vi "NumIntegrate_Rkdp_impl.vi"(4 "MaxTruncError":dbl, 5 "Func_X_U_Extra":T1, 6 "dT_Remaining":dbl, 7 "PassedData":variant, 8 "InitialH":dbl, 10 "U":T2, 11 "X":T2) -> (0 "Error":bool, 1 "IterationCount":i32, 2 "H":dbl, 3 "NewX":T2)   [LabVIEW 2019, in "Trajectory_Library.lvlib"]
doc: "Implements one loop of RKDP. This takes an initial state, dt guess, and max truncation error, and returns a new x and the dt over which that x was updated. This should be called until there is no dt remaining.\n\nThis is an INTERNAL FUNCTION AND SHOULD NOT BE CALLED DIRECTLY.\n\n\n\nInputs:\n - Func_X_U_Extra -- A strictly typed LabVIEW reference to a function to integrate as a function of matrix X, U, and the extra passed data\n - PassedData -- This is a variant that can be used to pass additional data to the function if needed. The data must be packed into the variant in the specific way expected by the function.\n - X -- The initial value of x.\n - U -- The value u held constant over the integration period.\n - InitialH -- The initial dt guess. This is refined to clamp truncation error to the specified max.\n - dT_Remaining -- How much time is left to integrate over. Used to clamp h.\n - Max TruncError -- The max truncation error acceptable. Usually a small number like 1e-6.\n\nOutputs:\n - New X -- the integration of dx/dt = f(x, u) for dt\n - H -- \n - Iteration count -- How many times this routine looped to achieve the desired error tolerance\n - Error -- If TRUE, an error occured."
uses:
  Trajectory_Library.lvlib
  <vilib>/Analysis/Matrix/Datatypes/RealMatrix.ctl
  TypeDef/CALLBACK_FUNC_TYPE.ctl
  NumIntegrate_Rkdp_Func_B1.vi
  NumIntegrate_Rkdp_Func_B2.vi
  <vilib>/Analysis/_algsub.llb/Matrix Norm.vi
  <vilib>/Analysis/_algsub.llb/Real Matrix Norm.vi
  <vilib>/Analysis/Matrix/Numeric/Multiply/Multiply - RM,R.vi
  <vilib>/Analysis/Matrix/Numeric/Add/Add - RM,RM.vi
  <vilib>/Analysis/Matrix/NI_Matrix.lvlib
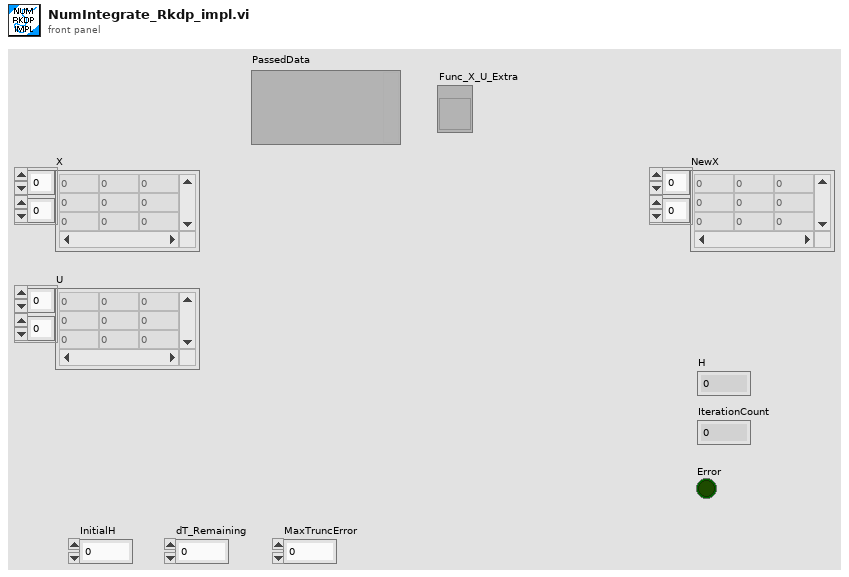
[diagram p1: front panel]
types:
  T1 = typedef "Trajectory_Library.lvlib/CALLBACK_FUNC_TYPE.ctl" = refnum<vi>
  T2 = typedef "NI_Matrix.lvlib/RealMatrix.ctl" = dbl[][]
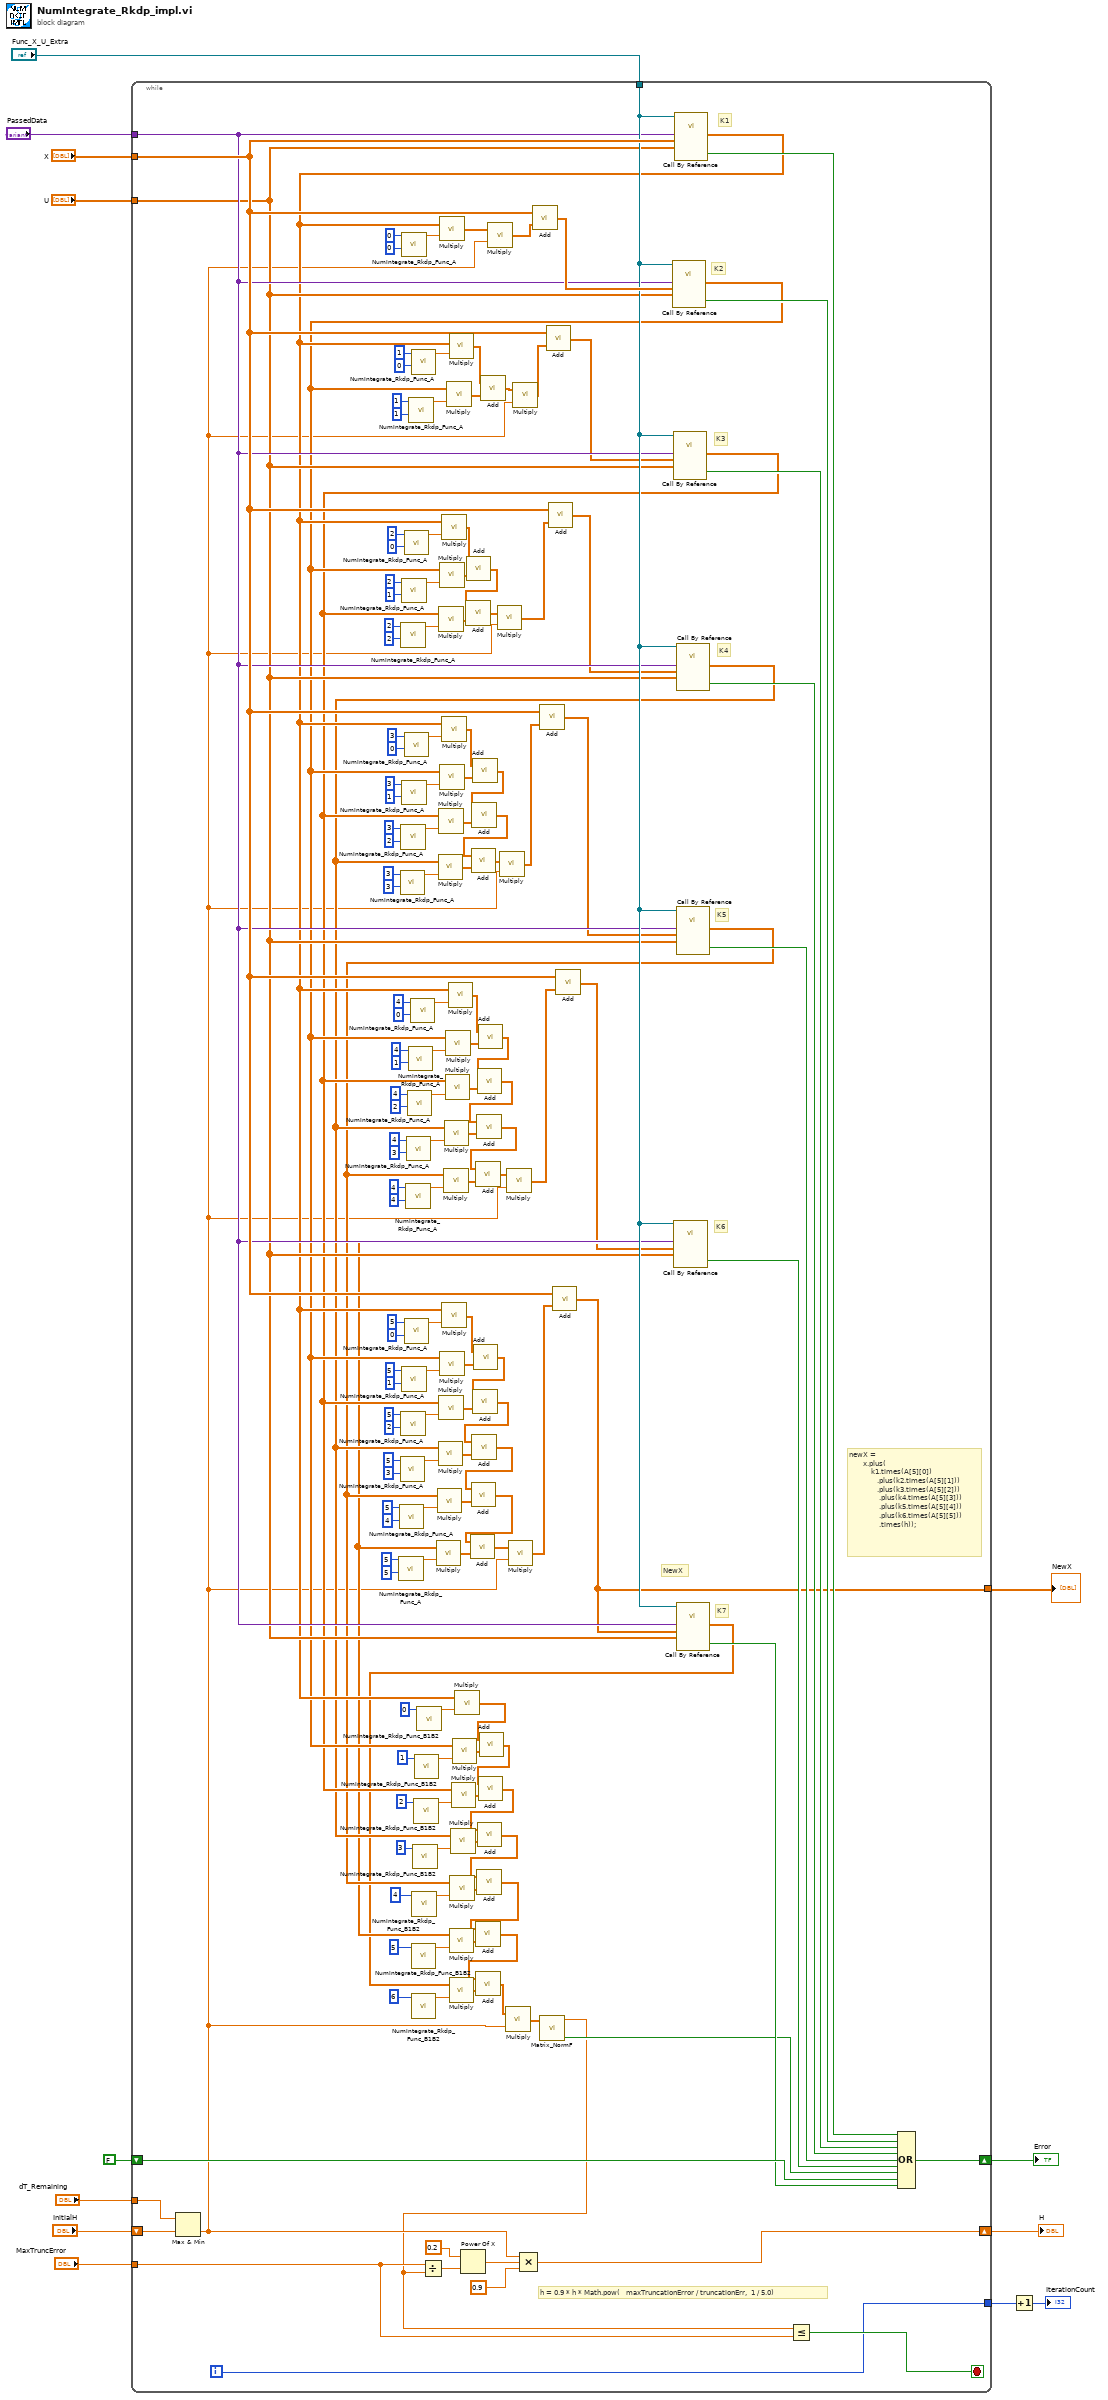
[diagram p0: block diagram]
diagram:
  n1 = while {
    tunnel: "PassedData" -> [w54]
    shift-right: [w76] -> w8
    shift-left: "InitialH" -> [w75]
    tunnel: "X" -> [w70]
    tunnel: "U" -> [w53]
    tunnel: "MaxTruncError" -> [w73]
    tunnel: "dT_Remaining" -> [w74]
    tunnel: [w24] -> w5
    tunnel: [w71] -> w7
    tunnel: "Func_X_U_Extra" -> [w55]
    shift-right: [w62] -> w1
    shift-left: FALSE -> [w69]
    i -> [w71]
    stop <- w72 stop-if-true
    # "K7"
    # "newX =\n       x.plus(\n           k1.times(A[5][0])\n              .plus(k2.times(A[5][1]))\n              .plus(k3.times(A[5][2]))\n               .plus(k4.times(A[5][3]))\n               .plus(k5.times(A[5][4]))\n               .plus(k6.times(A[5][5]))\n               .times(h));"
    # "K6"
    # "K5"
    # "K4"
    # "K3"
    # "K2"
    # "K1"
    # "h = 0.9 * h * Math.pow(   maxTruncationError / truncationErr,  1 / 5.0)"
    # "NewX"
    n2 = Max & Min(x=w74, y=w75) -> (min(x,y)=w17:dbl)  [unwired: 1 out]
    n3 = call "NumIntegrate_Rkdp_Func_A.vi"("Col"=5, "Row"=5) -> ("RKDP_A"=w106:dbl)  [unwired: 9 in]
    n4 = call "NumIntegrate_Rkdp_Func_A.vi"("Col"=4, "Row"=5) -> ("RKDP_A"=w110:dbl)  [unwired: 9 in]
    n5 = call "NumIntegrate_Rkdp_Func_A.vi"("Col"=3, "Row"=3) -> ("RKDP_A"=w150:dbl)  [unwired: 9 in]
    n6 = call "NumIntegrate_Rkdp_Func_A.vi"("Col"=3, "Row"=5) -> ("RKDP_A"=w114:dbl)  [unwired: 9 in]
    n7 = call "NumIntegrate_Rkdp_Func_A.vi"("Col"=2, "Row"=2) -> ("RKDP_A"=w167:dbl)  [unwired: 9 in]
    n8 = call "NumIntegrate_Rkdp_Func_A.vi"("Col"=2, "Row"=3) -> ("RKDP_A"=w155:dbl)  [unwired: 9 in]
    n9 = call "NumIntegrate_Rkdp_Func_A.vi"("Col"=2, "Row"=5) -> ("RKDP_A"=w118:dbl)  [unwired: 9 in]
    n10 = call "NumIntegrate_Rkdp_Func_A.vi"("Col"=0, "Row"=0) -> ("RKDP_A"=w185:dbl)  [unwired: 9 in]
    n11 = call "NumIntegrate_Rkdp_Func_A.vi"("Col"=1, "Row"=2) -> ("RKDP_A"=w171:dbl)  [unwired: 9 in]
    n12 = call "NumIntegrate_Rkdp_Func_A.vi"("Col"=1, "Row"=3) -> ("RKDP_A"=w159:dbl)  [unwired: 9 in]
    n13 = call "NumIntegrate_Rkdp_Func_A.vi"("Col"=1, "Row"=5) -> ("RKDP_A"=w121:dbl)  [unwired: 9 in]
    n14 = call "NumIntegrate_Rkdp_Func_A.vi"("Col"=0, "Row"=2) -> ("RKDP_A"=w174:dbl)  [unwired: 9 in]
    n15 = call "NumIntegrate_Rkdp_Func_A.vi"("Col"=0, "Row"=3) -> ("RKDP_A"=w162:dbl)  [unwired: 9 in]
    n16 = call "NumIntegrate_Rkdp_Func_A.vi"("Col"=0, "Row"=5) -> ("RKDP_A"=w123:dbl)  [unwired: 9 in]
    n17 = call "NumIntegrate_Rkdp_Func_A.vi"("Col"=4, "Row"=4) -> ("RKDP_A"=w128:dbl)  [unwired: 9 in]
    n18 = call "NumIntegrate_Rkdp_Func_A.vi"("Col"=3, "Row"=4) -> ("RKDP_A"=w133:dbl)  [unwired: 9 in]
    n19 = call "NumIntegrate_Rkdp_Func_A.vi"("Col"=2, "Row"=4) -> ("RKDP_A"=w138:dbl)  [unwired: 9 in]
    n20 = call "NumIntegrate_Rkdp_Func_A.vi"("Col"=1, "Row"=4) -> ("RKDP_A"=w142:dbl)  [unwired: 9 in]
    n21 = call "NumIntegrate_Rkdp_Func_A.vi"("Col"=1, "Row"=1) -> ("RKDP_A"=w178:dbl)  [unwired: 9 in]
    n22 = call "NumIntegrate_Rkdp_Func_A.vi"("Col"=0, "Row"=4) -> ("RKDP_A"=w145:dbl)  [unwired: 9 in]
    n23 = call "NumIntegrate_Rkdp_Func_A.vi"("Col"=0, "Row"=1) -> ("RKDP_A"=w181:dbl)  [unwired: 9 in]
    n24 = call "NumIntegrate_Rkdp_Func_B1B2.vi"("Index"=5 ("Row")) -> ("RKDP_B1-B2"=w85:dbl)  [unwired: 10 in]
    n25 = call "NumIntegrate_Rkdp_Func_B1B2.vi"("Index"=6 ("Row")) -> ("RKDP_B1-B2"=w23:dbl)  [unwired: 10 in]
    n26 = call "NumIntegrate_Rkdp_Func_B1B2.vi"("Index"=4 ("Row")) -> ("RKDP_B1-B2"=w89:dbl)  [unwired: 10 in]
    n27 = call "NumIntegrate_Rkdp_Func_B1B2.vi"("Index"=3 ("Row")) -> ("RKDP_B1-B2"=w93:dbl)  [unwired: 10 in]
    n28 = call "NumIntegrate_Rkdp_Func_B1B2.vi"("Index"=2 ("Row")) -> ("RKDP_B1-B2"=w97:dbl)  [unwired: 10 in]
    n29 = call "NumIntegrate_Rkdp_Func_B1B2.vi"("Index"=1 ("Row")) -> ("RKDP_B1-B2"=w100:dbl)  [unwired: 10 in]
    n30 = call "NumIntegrate_Rkdp_Func_B1B2.vi"("Index"=0 ("Row")) -> ("RKDP_B1-B2"=w102:dbl)  [unwired: 10 in]
    n31 = call-by-ref "?"(reference=w55, "U"=w53, "X"=w70, "Variant"=w54) -> ("Error"=w63:bool, "NewX"=w51:T2)  [unwired: 8 in, 2 out]
    n32 = call-poly <vilib>:"Multiply.vi"("Real Scalar c"=w185, "Real Matrix A"=w51) -> ("A * c"=w45:T2)
    n33 = call-poly <vilib>:"Multiply.vi"("Real Scalar c"=w174, "Real Matrix A"=w51) -> ("A * c"=w39:T2)
    n34 = call-poly <vilib>:"Multiply.vi"("Real Scalar c"=w162, "Real Matrix A"=w51) -> ("A * c"=w35:T2)
    n35 = call-poly <vilib>:"Multiply.vi"("Real Scalar c"=w123, "Real Matrix A"=w51) -> ("A * c"=w27:T2)
    n36 = call-poly <vilib>:"Multiply.vi"("Real Scalar c"=w145, "Real Matrix A"=w51) -> ("A * c"=w31:T2)
    n37 = call-poly <vilib>:"Multiply.vi"("Real Scalar c"=w181, "Real Matrix A"=w51) -> ("A * c"=w43:T2)
    n38 = call-poly <vilib>:"Multiply.vi"("Real Scalar c"=w102, "Real Matrix A"=w51) -> ("A * c"=w81:T2)
    n39 = call-poly <vilib>:"Multiply.vi"("Real Scalar c"=w17, "Real Matrix A"=w45) -> ("A * c"=w44:T2)
    n40 = call-poly <vilib>:"Add.vi"("Real Matrix B"=w44, "Real Matrix A"=w70) -> ("A + B"=w184:T2)
    n41 = call-by-ref "?"(reference=w55, "U"=w53, "X"=w184, "Variant"=w54) -> ("Error"=w64:bool, "NewX"=w50:T2)  [unwired: 8 in, 2 out]
    n42 = call-poly <vilib>:"Multiply.vi"("Real Scalar c"=w171, "Real Matrix A"=w50) -> ("A * c"=w170:T2)
    n43 = call-poly <vilib>:"Multiply.vi"("Real Scalar c"=w159, "Real Matrix A"=w50) -> ("A * c"=w158:T2)
    n44 = call-poly <vilib>:"Multiply.vi"("Real Scalar c"=w121, "Real Matrix A"=w50) -> ("A * c"=w120:T2)
    n45 = call-poly <vilib>:"Multiply.vi"("Real Scalar c"=w142, "Real Matrix A"=w50) -> ("A * c"=w141:T2)
    n46 = call-poly <vilib>:"Multiply.vi"("Real Scalar c"=w178, "Real Matrix A"=w50) -> ("A * c"=w177:T2)
    n47 = call-poly <vilib>:"Multiply.vi"("Real Scalar c"=w100, "Real Matrix A"=w50) -> ("A * c"=w99:T2)
    n48 = call-poly <vilib>:"Add.vi"("Real Matrix B"=w170, "Real Matrix A"=w39) -> ("A + B"=w163:T2)
    n49 = call-poly <vilib>:"Add.vi"("Real Matrix B"=w158, "Real Matrix A"=w35) -> ("A + B"=w151:T2)
    n50 = call-poly <vilib>:"Add.vi"("Real Matrix B"=w120, "Real Matrix A"=w27) -> ("A + B"=w115:T2)
    n51 = call-poly <vilib>:"Add.vi"("Real Matrix B"=w141, "Real Matrix A"=w31) -> ("A + B"=w134:T2)
    n52 = call-poly <vilib>:"Add.vi"("Real Matrix B"=w99, "Real Matrix A"=w81) -> ("A + B"=w94:T2)
    n53 = call-poly <vilib>:"Add.vi"("Real Matrix B"=w177, "Real Matrix A"=w43) -> ("A + B"=w42:T2)
    n54 = call-poly <vilib>:"Multiply.vi"("Real Scalar c"=w17, "Real Matrix A"=w42) -> ("A * c"=w41:T2)
    n55 = call-poly <vilib>:"Add.vi"("Real Matrix B"=w41, "Real Matrix A"=w70) -> ("A + B"=w40:T2)
    n56 = call-by-ref "?"(reference=w55, "U"=w53, "X"=w40, "Variant"=w54) -> ("Error"=w65:bool, "NewX"=w49:T2)  [unwired: 8 in, 2 out]
    n57 = call-poly <vilib>:"Multiply.vi"("Real Scalar c"=w167, "Real Matrix A"=w49) -> ("A * c"=w166:T2)
    n58 = call-poly <vilib>:"Multiply.vi"("Real Scalar c"=w155, "Real Matrix A"=w49) -> ("A * c"=w154:T2)
    n59 = call-poly <vilib>:"Multiply.vi"("Real Scalar c"=w118, "Real Matrix A"=w49) -> ("A * c"=w117:T2)
    n60 = call-poly <vilib>:"Multiply.vi"("Real Scalar c"=w138, "Real Matrix A"=w49) -> ("A * c"=w137:T2)
    n61 = call-poly <vilib>:"Multiply.vi"("Real Scalar c"=w97, "Real Matrix A"=w49) -> ("A * c"=w96:T2)
    n62 = call-poly <vilib>:"Add.vi"("Real Matrix B"=w166, "Real Matrix A"=w163) -> ("A + B"=w38:T2)
    n63 = call-poly <vilib>:"Add.vi"("Real Matrix B"=w154, "Real Matrix A"=w151) -> ("A + B"=w146:T2)
    n64 = call-poly <vilib>:"Add.vi"("Real Matrix B"=w117, "Real Matrix A"=w115) -> ("A + B"=w111:T2)
    n65 = call-poly <vilib>:"Add.vi"("Real Matrix B"=w137, "Real Matrix A"=w134) -> ("A + B"=w129:T2)
    n66 = call-poly <vilib>:"Add.vi"("Real Matrix B"=w96, "Real Matrix A"=w94) -> ("A + B"=w90:T2)
    n67 = call-poly <vilib>:"Multiply.vi"("Real Scalar c"=w17, "Real Matrix A"=w38) -> ("A * c"=w37:T2)
    n68 = call-poly <vilib>:"Add.vi"("Real Matrix B"=w37, "Real Matrix A"=w70) -> ("A + B"=w36:T2)
    n69 = call-by-ref "?"(reference=w55, "U"=w53, "X"=w36, "Variant"=w54) -> ("Error"=w66:bool, "NewX"=w48:T2)  [unwired: 8 in, 2 out]
    n70 = call-poly <vilib>:"Multiply.vi"("Real Scalar c"=w150, "Real Matrix A"=w48) -> ("A * c"=w149:T2)
    n71 = call-poly <vilib>:"Multiply.vi"("Real Scalar c"=w114, "Real Matrix A"=w48) -> ("A * c"=w113:T2)
    n72 = call-poly <vilib>:"Multiply.vi"("Real Scalar c"=w133, "Real Matrix A"=w48) -> ("A * c"=w132:T2)
    n73 = call-poly <vilib>:"Multiply.vi"("Real Scalar c"=w93, "Real Matrix A"=w48) -> ("A * c"=w92:T2)
    n74 = call-poly <vilib>:"Add.vi"("Real Matrix B"=w149, "Real Matrix A"=w146) -> ("A + B"=w34:T2)
    n75 = call-poly <vilib>:"Add.vi"("Real Matrix B"=w113, "Real Matrix A"=w111) -> ("A + B"=w107:T2)
    n76 = call-poly <vilib>:"Add.vi"("Real Matrix B"=w132, "Real Matrix A"=w129) -> ("A + B"=w124:T2)
    n77 = call-poly <vilib>:"Add.vi"("Real Matrix B"=w92, "Real Matrix A"=w90) -> ("A + B"=w86:T2)
    n78 = call-poly <vilib>:"Multiply.vi"("Real Scalar c"=w17, "Real Matrix A"=w34) -> ("A * c"=w33:T2)
    n79 = call-poly <vilib>:"Add.vi"("Real Matrix B"=w33, "Real Matrix A"=w70) -> ("A + B"=w32:T2)
    n80 = call-by-ref "?"(reference=w55, "U"=w53, "X"=w32, "Variant"=w54) -> ("Error"=w67:bool, "NewX"=w47:T2)  [unwired: 8 in, 2 out]
    n81 = call-poly <vilib>:"Multiply.vi"("Real Scalar c"=w110, "Real Matrix A"=w47) -> ("A * c"=w109:T2)
    n82 = call-poly <vilib>:"Multiply.vi"("Real Scalar c"=w128, "Real Matrix A"=w47) -> ("A * c"=w127:T2)
    n83 = call-poly <vilib>:"Multiply.vi"("Real Scalar c"=w89, "Real Matrix A"=w47) -> ("A * c"=w88:T2)
    n84 = call-poly <vilib>:"Add.vi"("Real Matrix B"=w109, "Real Matrix A"=w107) -> ("A + B"=w103:T2)
    n85 = call-poly <vilib>:"Add.vi"("Real Matrix B"=w127, "Real Matrix A"=w124) -> ("A + B"=w30:T2)
    n86 = call-poly <vilib>:"Add.vi"("Real Matrix B"=w88, "Real Matrix A"=w86) -> ("A + B"=w82:T2)
    n87 = call-poly <vilib>:"Multiply.vi"("Real Scalar c"=w17, "Real Matrix A"=w30) -> ("A * c"=w29:T2)
    n88 = call-poly <vilib>:"Add.vi"("Real Matrix B"=w29, "Real Matrix A"=w70) -> ("A + B"=w28:T2)
    n89 = call-by-ref "?"(reference=w55, "U"=w53, "X"=w28, "Variant"=w54) -> ("Error"=w68:bool, "NewX"=w46:T2)  [unwired: 8 in, 2 out]
    n90 = call-poly <vilib>:"Multiply.vi"("Real Scalar c"=w106, "Real Matrix A"=w46) -> ("A * c"=w105:T2)
    n91 = call-poly <vilib>:"Multiply.vi"("Real Scalar c"=w85, "Real Matrix A"=w46) -> ("A * c"=w84:T2)
    n92 = call-poly <vilib>:"Add.vi"("Real Matrix B"=w105, "Real Matrix A"=w103) -> ("A + B"=w26:T2)
    n93 = call-poly <vilib>:"Add.vi"("Real Matrix B"=w84, "Real Matrix A"=w82) -> ("A + B"=w20:T2)
    n94 = call-poly <vilib>:"Multiply.vi"("Real Scalar c"=w17, "Real Matrix A"=w26) -> ("A * c"=w25:T2)
    n95 = call-poly <vilib>:"Add.vi"("Real Matrix B"=w25, "Real Matrix A"=w70) -> ("A + B"=w24:T2)
    n96 = call-by-ref "?"(reference=w55, "U"=w53, "X"=w24, "Variant"=w54) -> ("Error"=w52:bool, "NewX"=w19:T2)  [unwired: 8 in, 2 out]
    n97 = call-poly <vilib>:"Multiply.vi"("Real Scalar c"=w23, "Real Matrix A"=w19) -> ("A * c"=w22:T2)
    n98 = call-poly <vilib>:"Add.vi"("Real Matrix B"=w22, "Real Matrix A"=w20) -> ("A + B"=w18:T2)
    n99 = call-poly <vilib>:"Multiply.vi"("Real Scalar c"=w17, "Real Matrix A"=w18) -> ("A * c"=w16:T2)
    n100 = call "Matrix_NormF.vi"("input matrix"=w16) -> ("Error"=w15:bool, "normF"=w14:dbl)  [unwired: 9 in]
    n101 = Divide(x=w73, y=w14) -> (x/y=w79:dbl)
    n102 = Power Of X(1:w79, 2:0.2 ("x")) -> (0:w78:dbl)
    n103 = Compound Arithmetic op=MULTIPLY(w17, w78, 0.9 ("value")) -> (w76:dbl)
    n104 = Less Or Equal?(x=w14, y=w73) -> (x <= y?=w72:bool)
    n105 = Compound Arithmetic op=OR(w63, w64, w65, w66, w67, w68, w15, w69, w52) -> (w62:bool)
  }
  "NewX" <- w5
  "H" <- w8
  "Error" <- w1
  n106 = Increment(x=w7) -> (x+1=→"IterationCount":i32)
